vi "Teleop.vi"(10 "Match Info":T2={"Autonomous Elapsed Seconds"=0.0, "TeleOp Elapsed Seconds"=0.0, "Disabled Elapsed Seconds"=0.0, "Visited Autonomous"=FALSE, "Visited TeleOp"=FALSE, "Visited Disabled"=FALSE, "Autonomous Settings"={"Autonomous Style"=enum."Independent", "VI Refnum"=refnum}}, 11 "Call Context":T3) -> ()   [LabVIEW 2016]
doc: "This VI is called for each TeleOp packet received from the DS where the robot is not disabled. It is often used to read from the joysticks and update I/O or to update setpoints for timed control loops. It should complete and return within 20 milliseconds or it may miss DS packets."
uses:
  <vilib>/Rock Robotics/WPI/DriverStation/WPI_DriverStationDerivedRobotMode.ctl
  <vilib>/Rock Robotics/WPI/DriverStation/WPI_DriverStationMatch Info.ctl
  Robot Global Data.vi
  <vilib>/Rock Robotics/WPI/Utilities/WPI_GetSetVariantRefNum.vi
  <vilib>/Rock Robotics/WPI/Solenoid/Deprecated/WPI_SolenoidSetBool.vi
  <vilib>/Rock Robotics/Network Tables/NT Write Number.vi
  <vilib>/Rock Robotics/Network Tables/NT Write Boolean.vi
  <vilib>/addons/control/pid/pid.llb/PID (DBL).vi
  navX Library v2/navX Library v2.lvlib
  <vilib>/addons/control/pid/NI_PID_pid.lvlib
panel:
  in  "MOE":dbl=25.0 format="%#_13g"
  in  "Center":dbl=180.0 format="%#_13g"
  out "out left":dbl
  out "out right":dbl
  in  "Pid Factor":dbl=8400.0
  in  "Mode":bool=TRUE
  in  "output range":cluster{"output high":dbl, "output low":dbl}={"output high"=1.0, "output low"=-1.0} {"output low" format="%.2f"; "output high" format="%.2f"}
  in  "PID gains":T1={"proportional gain (Kc)"=0.00021, "integral time (Ti, min)"=15.0, "derivative time (Td, min)"=0.0} {"derivative time (Td, min)" format="%.6f"; "integral time (Ti, min)" format="%.6f"; "proportional gain (Kc)" format="%.6f"}
  out "Left":dbl(graph)
  out "Right":dbl(graph)
  out "Encoder Right":dbl(graph)
  out "Encoder Left":dbl(graph)
  in  "Speed":dbl=0.45 format="%#_13g"
  out "Out Left":dbl(graph)
  out "Out Right":dbl(graph)
  out "Shooter":cluster{"Sensor Velocity":dbl, dbl, dbl}(graph)
  in  "ShooterRPM":dbl
  in  "P":dbl=0.5 format="%#_13g"
  in  "I":dbl format="%#_13g"
  in  "D":dbl format="%#_13g"
  in  "F":dbl=0.005212 format="%#_13g"
  in  "I Zone":dbl format="%#_13g"
  in  "Ramp Rate":dbl format="%#_13g"
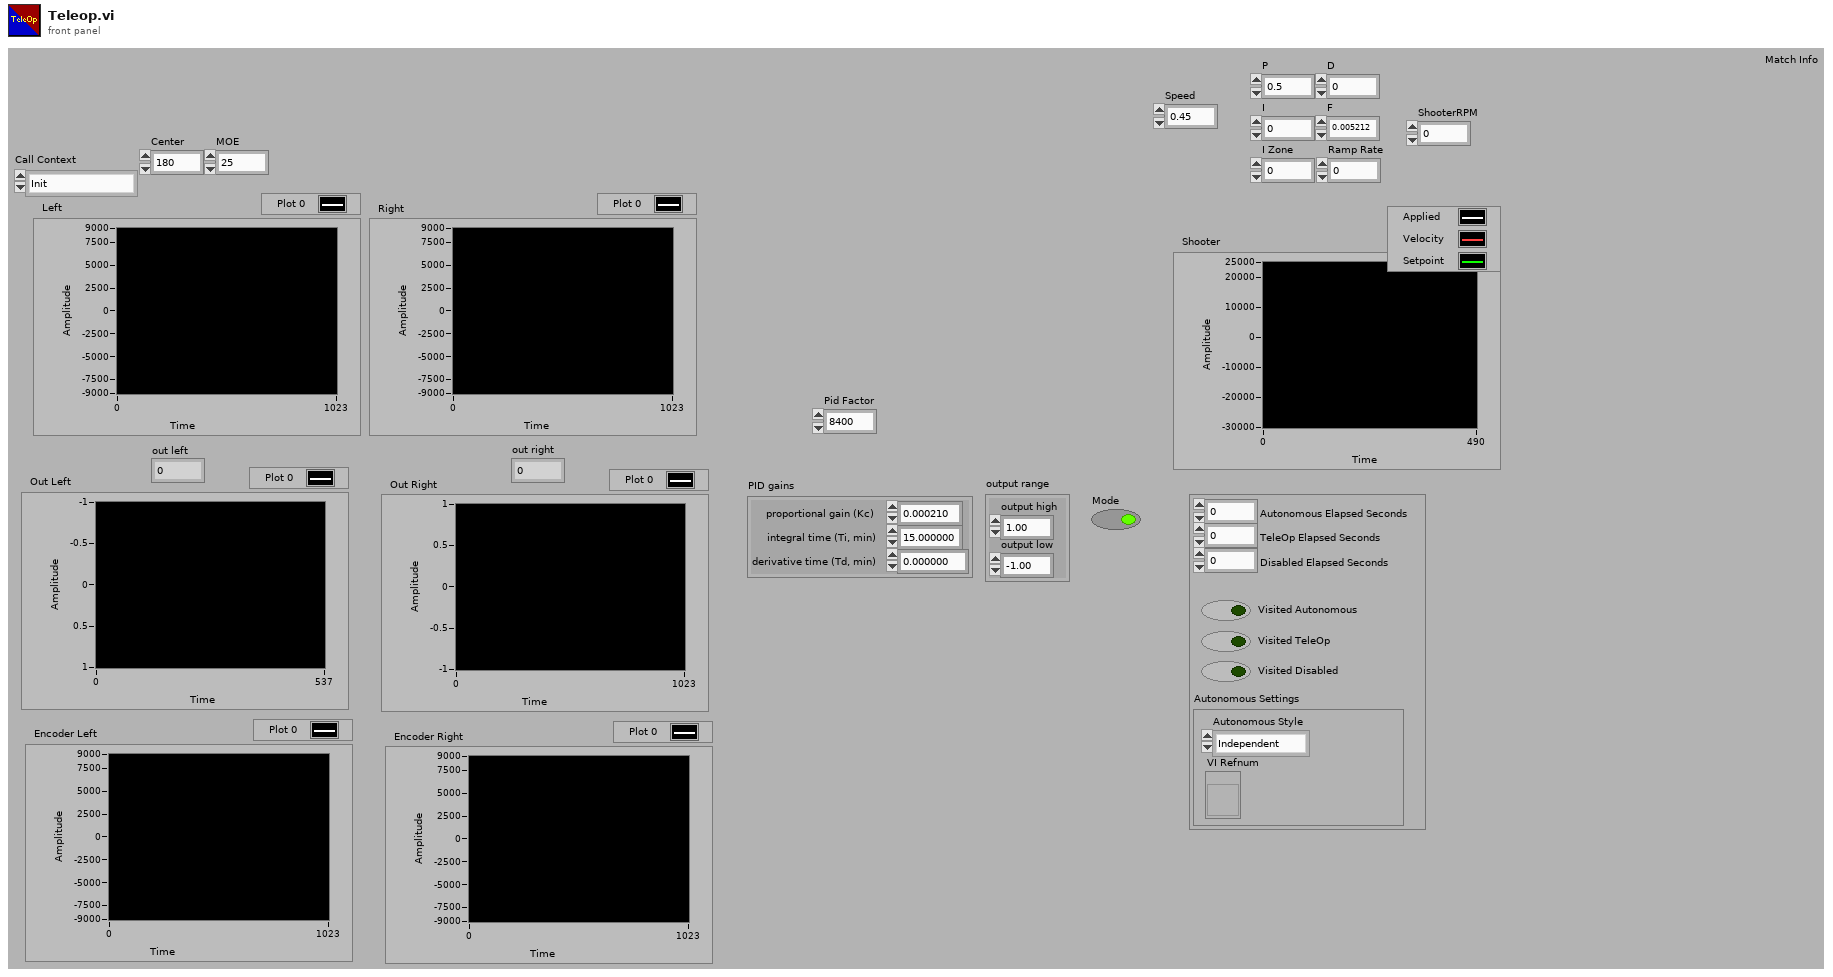
[diagram p1: front panel]
types:
  T1 = cluster{"proportional gain (Kc)":dbl, "integral time (Ti, min)":dbl, "derivative time (Td, min)":dbl}
  T2 = typedef "WPI_DriverStationMatch Info.ctl" = cluster{"Autonomous Elapsed Seconds":dbl, "TeleOp Elapsed Seconds":dbl, "Disabled Elapsed Seconds":dbl, "Visited Autonomous":bool, "Visited TeleOp":bool, "Visited Disabled":bool, "Autonomous Settings":cluster{"Autonomous Style":enum16{"Iterative", "Independent"}, "VI Refnum":refnum<vi>}}
  T3 = typedef "WPI_DriverStationDerivedRobotMode.ctl" = enum16{"Init", "Execute", "Stop"}
  T4 = typedef "WPI_SolenoidDevRef.ctl" = cluster{"DevStatus":errorcluster, "Pneumatics Control Module":u8, "Forward Solenoid Channel":T5, "Reverse Solenoid Channel":T5}
  T5 = typedef "WPI_SolenoidChannel.ctl" = enum8{"Solenoid 0", "Solenoid 1", "Solenoid 2", "Solenoid 3", "Solenoid 4", "Solenoid 5", "Solenoid 6", "Solenoid 7", "Invalid"}
  T6 = typedef "WPI_JoystickDevRef.ctl" = cluster{"Device":T7}
  T7 = typedef "WPI_JoystickDeviceEnum.ctl" = enum16{"USB 0", "USB 1", "USB 2", "USB 3", "USB 4", "USB 5"}
  T8 = cluster{"Buttons[0]":bool, "Buttons[1]":bool, "Buttons[2]":bool, "Buttons[3]":bool, "Buttons[4]":bool, "Buttons[5]":bool, "Buttons[6]":bool, "Buttons[7]":bool, "Buttons[8]":bool}
  T9 = cluster{"Axes[0]":dbl, "Axes[1]":dbl, "Axes[2]":dbl, "Axes[3]":dbl, "Axes[4]":dbl, "Axes[5]":dbl, "Axes[6]":dbl, "Axes[7]":dbl, "Axes[8]":dbl}
  T10 = typedef "navX Library v2.lvlib/Z900_navX_DeviceTypeDef.ctl" = cluster{"Interface":cluster{"Protocol":T11, "Update Rate (4Hz-100Hz)":u8, "navX Open TypeDef":variant}, "Notify Packet":refnum<notifier>, "Loop VI Refnum":refnum<vi>, "Ready to Close Occurrence Refnum":refnum<k4>}
  T11 = typedef "navX Library v2.lvlib/Z900_navX_ProtocolTypeDef.ctl" = enum16{"SERIAL", "I2C", "SPI"}
  T12 = cluster{"Velocity X":dbl, "Velocity Y":dbl, "Velocity Z":dbl, "Displacement X":dbl, "Displacement Y":dbl, "Displacement Z":dbl}
  T13 = cluster{"LinearAcceleration X":dbl, "LinearAcceleration Y":dbl, "LinearAcceleration Z":dbl}
  T14 = cluster{"Yaw":dbl, "Roll":dbl, "Pitch":dbl, "Heading":dbl, "Fused Heading":dbl}
  T15 = typedef "WPI_MotorControlDeviceRef.ctl" = cluster{"DeviceStatus":errorcluster, "Type":T16, "PWM":cluster{"PWM Channel":T17, "DeadBand":T18}, "CAN":cluster{"Device Number":u8, "SetOutput VI Ref":variant, "GetOutput VI Ref":variant, "Enable VI Ref":variant, "Disable VI Ref":variant, "Data":variant}, "Invert":bool}
  T16 = typedef "WPI_MotorControlType.ctl" = enum16{"PWM", "CAN"}
  T17 = typedef "FPGA_DIOPWMChannel.ctl" = enum8{"PWM 0", "PWM 1", "PWM 2", "PWM 3", "PWM 4", "PWM 5", "PWM 6", "PWM 7", "PWM 8", "PWM 9", "PWM MXP 0", "PWM MXP 1", "PWM MXP 2", "PWM MXP 3", "PWM MXP 4", "PWM MXP 5", "PWM MXP 6", "PWM MXP 7", "PWM MXP 8", "PWM MXP 9", "Invalid"}
  T18 = typedef "WPI_PWMDeadband.ctl" = cluster{"Name":string, "maxPositivePwm":i32, "minPositivePwm":i32, "centerPwm":i32, "maxNegativePwm":i32, "minNegativePwm":i32, "angularRange":u16}
  T19 = typedef "WPI_CANTalonSRX_GlobalStatus.ctl" = cluster{"Applied Throttle":dbl, "Module Enabled":bool, "CAN Error":errorcluster, "Closed Loop Error":dbl, "Forward Limit Switch Closed":bool, "Reverse Limit Switch Closed":bool, "Sensor Position":dbl, "Sensor Velocity":dbl, "Current":dbl, "Sticky Fault - Over Temp":bool, "Sticky Fault - Under Voltage":bool, "Sticky Fault - Forward Limit":bool, "Sticky Fault - Reverse Limit":bool, "Sticky Fault - Forward Soft Limit":bool, "Sticky Fault - Reverse Soft Limit":bool, "Brake is Enabled":bool, "Encoder Position":dbl, "Encoder Velocity":dbl, "Encoder Index Count":dbl, "Encoder A Pin State":bool, "Encoder B Pin State":bool, "Encoder Index Pin State":bool, "Analog In":dbl, "Analog In Velocity":dbl, "Temperature (C)":dbl, "Battery Voltage":dbl, "Control 5 Is Supported":bool, "Current Profile Slot Select":dbl, "Pos Div 8":bool, "Vel Div 4":bool, "Pulse Width Position":i32, "Pulse Width Velocity":i32, "Pulse Width Rise To Rise (us)":i32, "Pulse Width Rise To Fall (us)":i32, "Mot Prof Active Is Under Run":bool, "Mot Prof Active Has Under Run":bool, "Mot Prof Active Is Last":bool, "Mot Prof Active Velocity Only":bool, "Mot Prof Active Is Valid":bool, "Mot Prof Buffer Is Full":bool, "Mot Prof Active Profile Slot Select":i32, "Mot Prof NextID":i32, "Mot Prof Count":i32, "Mot Prof Active Velocity":dbl, "Mot Prof Active Position":dbl, "Mot Prof Output Enable":i32}
  T20 = cluster{dbl, "Sensor Velocity":dbl, "ShooterRPM":dbl}
  T21 = typedef "WPI_EncoderDevRef.ctl" = cluster{"DevStatus":errorcluster, "EncoderIndex":T22, "CounterIndex":T23, "DistancePerCount":dbl, "Decoding Type":T24}
  T22 = typedef "FPGA_EncoderIdx.ctl" = enum8{"Enc 0", "Enc 1", "Enc 2", "Enc 3", "Enc 4", "Enc 5", "Enc 6", "Enc 7", "Invalid"}
  T23 = typedef "FPGA_CounterCtrSystemIndex.ctl" = enum8{"Ctr 0", "Ctr 1", "Ctr 2", "Ctr 3", "Ctr 4", "Ctr 5", "Ctr 6", "Ctr 7", "Invalid"}
  T24 = typedef "WPI_EncoderType.ctl" = enum16{"1x", "2x", "4x"}
  T25 = typedef "WPI_RobotDriveDevRef.ctl" = cluster{"DevStatus":errorcluster, "Motors[]":T15[], "Square Inputs":bool, "Max Output":dbl}
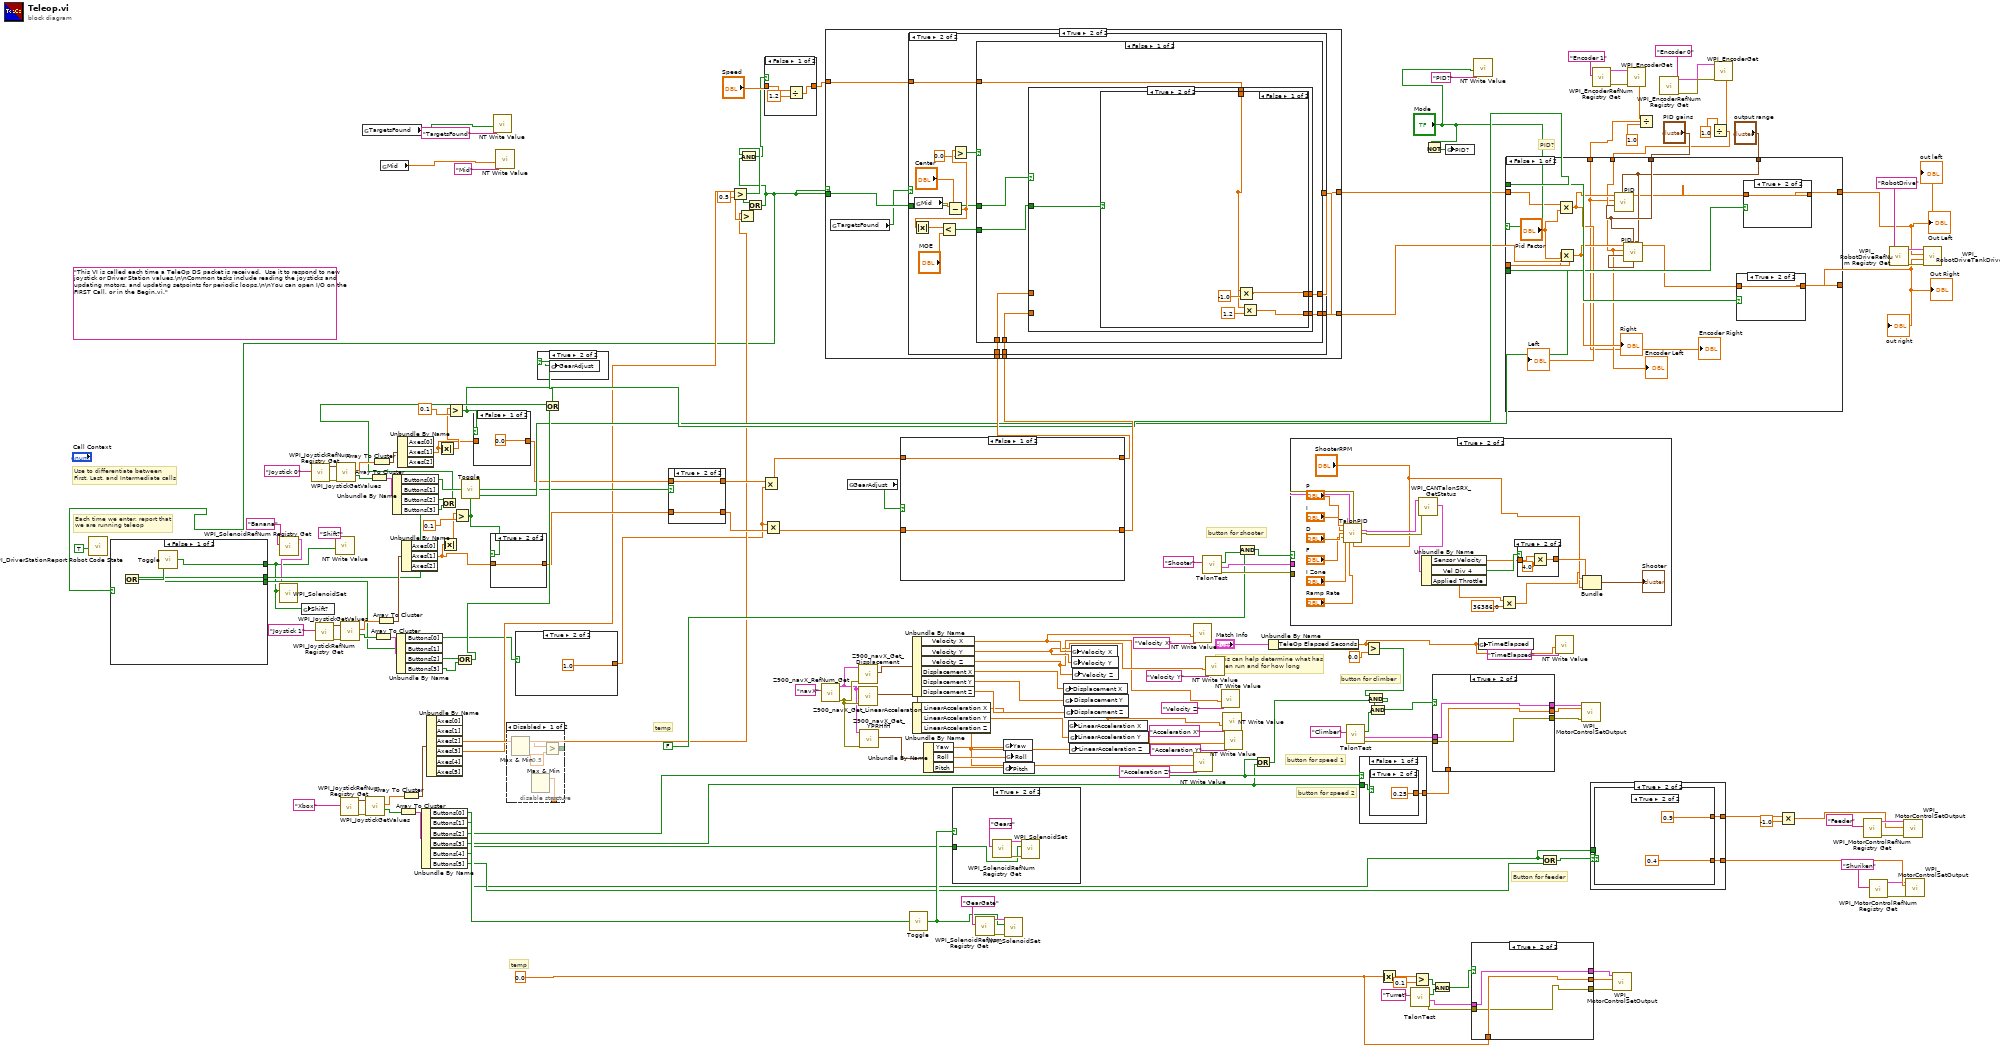
[diagram p0: block diagram]
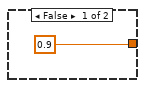
[diagram p2: hidden frame]
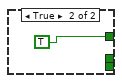
[diagram p3: hidden frame]
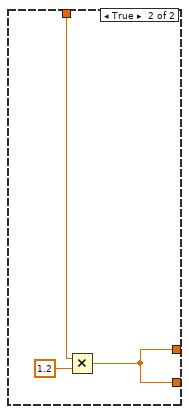
[diagram p8: hidden frame]
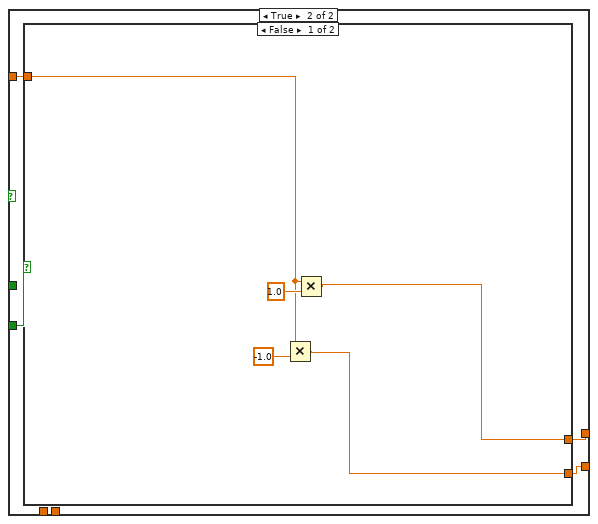
[diagram p9: hidden frame]
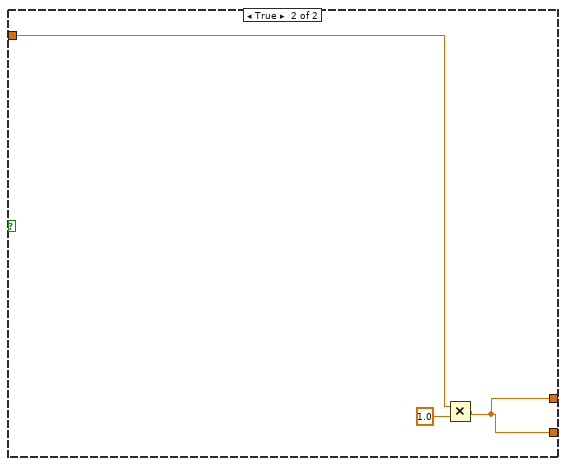
[diagram p10: hidden frame]
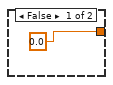
[diagram p11: hidden frame]
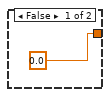
[diagram p12: hidden frame]
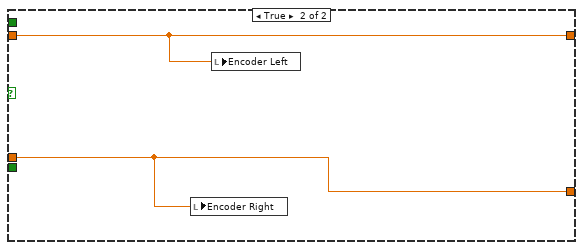
[diagram p13: hidden frame]
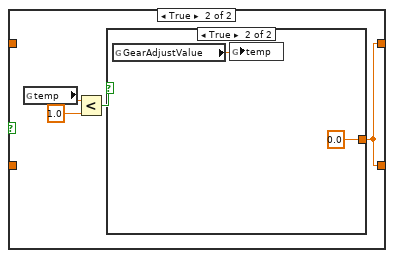
[diagram p16: hidden frame]
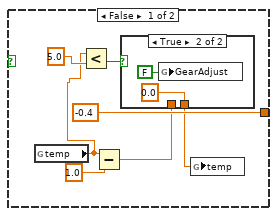
[diagram p17: hidden frame]
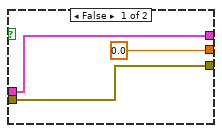
[diagram p19: hidden frame]
diagram:
  w38 = 0.5 ("y")
  w78 = 0.0
  (unwired) "This VI is called each time a TeleOp DS packet is received.  Use it to respond to new joystick or Driver Station values.\n\nCommon tasks include reading the joysticks and updating motors, and updating setpoints for periodic loops.\n\nYou can open I/O on the FIRST Call, or in the Begin.vi."
  # "PID?"
  # "temp"
  # "temp"
  # "Button for feeder"
  # "button for speed 2"
  # "button for speed 1"
  # "button for climber"
  # "button for shooter"
  # "Each time we enter, report that\nwe are running teleop"
  # "Use to differentiate between\nFirst, Last, and Intermediate calls"
  # "This can help determine what has\nbeen run and for how long"
  n1 = call <vilib>:"WPI_DriverStationReport Robot Code State.vi"("TeleOp"=TRUE ("Autonomous")) -> ()  [unwired: 10 in, 1 out]
  n2 = call <vilib>:"WPI_SolenoidRefNum Registry Get.vi"("refnum name"="Banana") -> ("SolenoidDevRef"=w8:T4)  [unwired: 9 in, 1 out]
  n3 = call <vilib>:"WPI_JoystickRefNum Registry Get.vi"("refnum name"="Joystick 0") -> ("error out"=w171:errorcluster, "JoystickDevRef"=w170:T6)  [unwired: 9 in]
  n4 = call <vilib>:"WPI_JoystickRefNum Registry Get.vi"("refnum name"="Joystick 1") -> ("error out"=w163:errorcluster, "JoystickDevRef"=w162:T6)  [unwired: 9 in]
  n5 = call <vilib>:"WPI_JoystickGetValues.vi"("error in (no error)"=w171, "JoystickDevRef"=w170) -> ("Buttons"=w167:bool[], "Axes"=w168:dbl[])  [unwired: 5 in, 3 out]
  n6 = call <vilib>:"WPI_JoystickRefNum Registry Get.vi"("refnum name"="Xbox") -> ("error out"=w125:errorcluster, "JoystickDevRef"=w124:T6)  [unwired: 9 in]
  n7 = call <vilib>:"WPI_JoystickGetValues.vi"("error in (no error)"=w163, "JoystickDevRef"=w162) -> ("Buttons"=w159:bool[], "Axes"=w160:dbl[])  [unwired: 5 in, 3 out]
  n8 = global read "Robot Global Data.vi" "TargetsFound"() -> (w12:bool)
  n9 = call <vilib>:"WPI_JoystickGetValues.vi"("error in (no error)"=w125, "JoystickDevRef"=w124) -> ("Buttons"=w121:bool[], "Axes"=w122:dbl[])  [unwired: 5 in, 3 out]
  n10 = Array To Cluster(array=w167) -> (cluster=w165:T8)
  n11 = Array To Cluster(array=w168) -> (cluster=w166:T9)
  n12 = Array To Cluster(array=w159) -> (cluster=w157:T8)
  n13 = Array To Cluster(array=w160) -> (cluster=w158:T9)
  n14 = global read "Robot Global Data.vi" "Mid"() -> (w10:dbl)
  n15 = Unbundle By Name(w165) -> ("Buttons[0]"=w151:bool, "Buttons[1]"=w41:bool, "Buttons[2]"=w84:bool, "Buttons[3]"=w83:bool)
  n16 = Unbundle By Name(w157) -> ("Buttons[0]"=w4:bool, "Buttons[1]"=w42:bool, "Buttons[2]"=w86:bool, "Buttons[3]"=w85:bool)
  n17 = Unbundle By Name(w166) -> ("Axes[1]"=w152:dbl)  [unwired: 2 out]
  n18 = Array To Cluster(array=w121) -> (cluster=w119:T8)
  n19 = Unbundle By Name(w158) -> ("Axes[1]"=w154:dbl)  [unwired: 2 out]
  n20 = Array To Cluster(array=w122) -> (cluster=w120:T9)
  n21 = Unbundle By Name(w119) -> ("Buttons[0]"=w118:bool, "Buttons[1]"=w117:bool, "Buttons[2]"=w116:bool, "Buttons[3]"=w115:bool, "Buttons[4]"=w112:bool, "Buttons[5]"=w113:bool)
  n22 = Unbundle By Name(w120) -> ("Axes[2]"=w32:dbl, "Axes[3]"=w31:dbl)  [unwired: 4 out]
  n23 = Absolute Value(x=w152) -> (abs(x)=w153:dbl)
  n24 = Or(x=w84, y=w83) -> (x .or. y?=w82:bool)
  n25 = Absolute Value(x=w154) -> (abs(x)=w155:dbl)
  n26 = Greater?(x=w153, y=0.1 ("x")) -> (0:w68:bool)
  n27 = Greater?(x=w155, y=0.1 ("x")) -> (0:w67:bool)
  n28 = Or(x=w86, y=w85) -> (x .or. y?=w81:bool)
  n29 = call "Toggle.vi"("Input"=w151) -> ("Output"=w62:bool)
  n30 = case shown="False" w68 {
    tunnel: w152 -> [_ w174]
    tunnel: [0.0 w174] -> w65
    frame False {
    }
    frame True {
    }
  }
  n31 = case shown="True" w67 {
    tunnel: w154 -> [_ w176]
    tunnel: [0.0 w176] -> w66
    frame False {
    }
    frame True {
    }
  }
  n32 = call-poly <vilib>:"NT Write Value.vi"("Boolean"=w12, "Name"="TargetsFound") -> ()  [unwired: 9 in, 1 out]
  n33 = call-poly <vilib>:"NT Write Value.vi"("Numeric"=w10, "Name"="Mid") -> ()  [unwired: 9 in, 1 out]
  n34 = disable-structure shown="Disabled" {
    disable-tunnel: [w178 _] -> _
    disable-tunnel: [w177 _] -> _
    frame Disabled {
      n35 = Max & Min() -> (max(x,y)=w180:dbl)  [unwired: 2 in, 1 out]
      n36 = Max & Min() -> (max(x,y)=w177:dbl)  [unwired: 2 in, 1 out]
      n37 = Greater?(x=w180, y=0.5) -> (0:w178:bool)
    }
    frame Enabled {
    }
  }
  n38 = case shown="True" w4 {
    tunnel: [0.9 1.0] -> w1
    frame False {
    }
    frame True {
    }
  }
  n39 = Or(x=w82, y=w81) -> (x .or. y?=w79:bool)
  n40 = case shown="True" w79 {
    selector: w79 -> [_ w183]
    frame False {
    }
    frame True {
      n41 = global write "Robot Global Data.vi" "GearAdjust"(w183) -> ()
    }
  }
  n42 = case shown="True" w62 {
    tunnel: w65 -> [w185 w190]
    tunnel: w66 -> [w184 w189]
    tunnel: [w188 w190] -> w64
    tunnel: [w187 w189] -> w63
    frame False {
      w186 = -1.0
      n43 = Multiply(x=w186, y=w185) -> (x*y=w187:dbl)
      n44 = Multiply(x=w184, y=w186) -> (x*y=w188:dbl)
    }
    frame True {
    }
  }
  n45 = Greater?(x=w31, y=w38) -> (0:w36:bool)
  n46 = Greater?(x=w32, y=w38) -> (0:w37:bool)
  n47 = Or(x=w36, y=w37) -> (x .or. y?=w7:bool)
  n48 = case shown="False" w7 {
    tunnel: w42 -> [w193 _]
    tunnel: w41 -> [w192 _]
    tunnel: [w191 TRUE] -> w5
    frame False {
      n49 = Or(x=w192, y=w193) -> (x .or. y?=w194:bool)
      n50 = call "Toggle.vi"("Input"=w194) -> ("Output"=w191:bool)
    }
    frame True {
    }
  }
  n51 = call-poly <vilib>:"WPI_SolenoidSet.vi"("Value"=w5, "SolenoidDevRef"=w8) -> ()  [unwired: 8 in, 2 out]
  n52 = global write "Robot Global Data.vi" "Shift?"(w5) -> ()
  n53 = call-poly <vilib>:"NT Write Value.vi"("Boolean"=w5, "Name"="Shift?") -> ()  [unwired: 9 in, 1 out]
  n54 = And(x=w36, y=w7) -> (x .and. y?=w33:bool)
  n55 = Multiply(x=w64, y=w1) -> (x*y=w3:dbl)
  n56 = case shown="False" w33 {
    tunnel: [w198 w199] -> w34
    tunnel: "Speed" -> [w197 w199]
    frame False {
      n57 = Divide(x=w197, y=1.2) -> (x/y=w198:dbl)
    }
    frame True {
    }
  }
  n58 = Multiply(x=w1, y=w63) -> (x*y=w2:dbl)
  n59 = call "Z900_navX_RefNum_Get.vi"("refnum name"="navX") -> ("error out"=w149:errorcluster, "navX Device"=w148:T10)  [unwired: 9 in]
  n60 = global read "Robot Global Data.vi" "GearAdjust"() -> (w80:bool)
  n61 = call "Z900_navX_Get_Displacement.vi"("error in (no error)"=w149, "navX Device"=w148) -> ("Displacement"=w145:T12)  [unwired: 6 in, 3 out]
  n62 = call "Z900_navX_Get_LinearAcceleration.vi"("error in (no error)"=w149, "navX Device"=w148) -> ("Linear Acceleration"=w146:T13)  [unwired: 6 in, 3 out]
  n63 = call "Z900_navX_Get_YPRHfH.vi"("error in (no error)"=w149, "navX Device"=w148) -> ("YRPHfH"=w147:T14)  [unwired: 6 in, 3 out]
  n64 = case shown="False" w80 {
    tunnel: w3 -> [w201 _]
    tunnel: w2 -> [w200 _]
    tunnel: [w201 w202] -> w73
    tunnel: [w200 w202] -> w72
    frame False {
    }
    frame True {
      n65 = global read "Robot Global Data.vi" "temp"() -> (w205:dbl)
      n66 = Less?(x=w205, y=1.0) -> (x < y?=w203:bool)
      n67 = case shown="True" w203 {
        tunnel: [-0.4 0.0] -> w202
        frame False {
          n68 = global read "Robot Global Data.vi" "temp"() -> (w208:dbl)
          n69 = Less?(x=w208, y=5.0 ("x")) -> (x < y?=w209:bool)
          n70 = Subtract(x=w208, y=1.0) -> (x-y=w206:dbl)
          n71 = case shown="True" w209 {
            tunnel: [w213 0.0] -> w207
            tunnel: w206 -> [w213 _]
            frame False {
            }
            frame True {
              n72 = global write "Robot Global Data.vi" "GearAdjust"(FALSE) -> ()
            }
          }
          n73 = global write "Robot Global Data.vi" "temp"(w207) -> ()
        }
        frame True {
          n74 = global read "Robot Global Data.vi" "GearAdjustValue"() -> (w217:dbl)
          n75 = global write "Robot Global Data.vi" "temp"(w217) -> ()
        }
      }
    }
  }
  n76 = case shown="True" w7 {
    tunnel: w73 -> [w219 w226]
    tunnel: w72 -> [w218 w225]
    tunnel: w7 -> [_ w224]
    tunnel: [w219 w220] -> w39
    tunnel: [w218 w221] -> w40
    tunnel: w34 -> [_ w222]
    frame False {
    }
    frame True {
      n77 = global read "Robot Global Data.vi" "TargetsFound"() -> (w223:bool)
      n78 = case shown="True" w223 {
        tunnel: w226 -> [w227 w237]
        tunnel: w225 -> [w228 w236]
        tunnel: [w227 w235] -> w220
        tunnel: [w228 w234] -> w221
        tunnel: w224 -> [_ w230]
        tunnel: w222 -> [_ w229]
        frame False {
        }
        frame True {
          n79 = global read "Robot Global Data.vi" "Mid"() -> (w242:dbl)
          n80 = Subtract(x=w242, y="Center") -> (x-y=w232:dbl)
          n81 = Absolute Value(x=w232) -> (abs(x)=w240:dbl)
          n82 = Less?(x=w240, y="MOE") -> (x < y?=w238:bool)
          n83 = Greater?(x=w232, y=0.0) -> (0:w233:bool)
          n84 = case shown="False" w233 {
            tunnel: w238 -> [w249 w267]
            tunnel: w237 -> [w248 _]
            tunnel: w236 -> [w247 _]
            tunnel: [w246 w265] -> w235
            tunnel: [w245 w266] -> w234
            tunnel: w230 -> [w244 _]
            tunnel: w229 -> [w243 w264]
            frame False {
              n85 = case shown="True" w244 {
                tunnel: w249 -> [_ w255]
                tunnel: w248 -> [w251 _]
                tunnel: w247 -> [w250 _]
                tunnel: [w251 w254] -> w245
                tunnel: [w250 w253] -> w246
                tunnel: w243 -> [_ w252]
                frame False {
                }
                frame True {
                  n86 = case shown="False" w255 {
                    tunnel: [w260 w263] -> w254
                    tunnel: [w258 w263] -> w253
                    tunnel: w252 -> [w256 w261]
                    frame False {
                      n87 = Multiply(x=w256, y=-1.0) -> (x*y=w260:dbl)
                      n88 = Multiply(x=w256, y=1.2) -> (x*y=w258:dbl)
                    }
                    frame True {
                      n89 = Multiply(x=w261, y=1.2) -> (x*y=w263:dbl)
                    }
                  }
                }
              }
            }
            frame True {
              n90 = case shown="False" w267 {
                tunnel: [w272 w275] -> w266
                tunnel: [w270 w275] -> w265
                tunnel: w264 -> [w268 w273]
                frame False {
                  n91 = Multiply(x=w268, y=-1.0) -> (x*y=w270:dbl)
                  n92 = Multiply(x=w268, y=1.0) -> (x*y=w272:dbl)
                }
                frame True {
                  n93 = Multiply(x=w273, y=1.0) -> (x*y=w275:dbl)
                }
              }
            }
          }
        }
      }
    }
  }
  n94 = call "Toggle.vi"("Input"=w118) -> ("Output"=w126:bool)
  n95 = Unbundle By Name(w145) -> ("Velocity X"=w19:dbl, "Velocity Y"=w18:dbl, "Velocity Z"=w17:dbl, "Displacement X"=w61:dbl, "Displacement Y"=w60:dbl, "Displacement Z"=w59:dbl)
  n96 = Unbundle By Name(w146) -> ("LinearAcceleration X"=w16:dbl, "LinearAcceleration Y"=w15:dbl, "LinearAcceleration Z"=w14:dbl)
  n97 = Unbundle By Name(w147) -> ("Yaw"=w58:dbl, "Roll"=w57:dbl, "Pitch"=w56:dbl)
  n98 = case shown="True" w126 {
    tunnel: w117 -> [_ w276]
    frame False {
    }
    frame True {
      n99 = call <vilib>:"WPI_SolenoidRefNum Registry Get.vi"("refnum name"="Gears") -> ("error out"=w279:errorcluster, "SolenoidDevRef"=w278:T4)  [unwired: 9 in]
      n100 = call-poly <vilib>:"WPI_SolenoidSet.vi"("error in (no error)"=w279, "Value"=w276, "SolenoidDevRef"=w278) -> ()  [unwired: 7 in, 2 out]
    }
  }
  n101 = call <vilib>:"WPI_SolenoidRefNum Registry Get.vi"("refnum name"="GearGate") -> ("error out"=w129:errorcluster, "SolenoidDevRef"=w128:T4)  [unwired: 9 in]
  n102 = global write "Robot Global Data.vi" "Pitch"(w56) -> ()
  n103 = global write "Robot Global Data.vi" "Yaw"(w58) -> ()
  n104 = call-poly <vilib>:"WPI_SolenoidSet.vi"("error in (no error)"=w129, "Value"=w126, "SolenoidDevRef"=w128) -> ()  [unwired: 7 in, 2 out]
  n105 = global write "Robot Global Data.vi" "Roll"(w57) -> ()
  n106 = global write "Robot Global Data.vi" "Displacement X"(w61) -> ()
  n107 = global write "Robot Global Data.vi" "Displacement Y"(w60) -> ()
  n108 = global write "Robot Global Data.vi" "Displacement Z"(w59) -> ()
  n109 = global write "Robot Global Data.vi" "LinearAcceleration X"(w16) -> ()
  n110 = global write "Robot Global Data.vi" "LinearAcceleration Y"(w15) -> ()
  n111 = global write "Robot Global Data.vi" "LinearAcceleration Z"(w14) -> ()
  n112 = global write "Robot Global Data.vi" "Velocity X"(w19) -> ()
  n113 = global write "Robot Global Data.vi" "Velocity Y"(w18) -> ()
  n114 = global write "Robot Global Data.vi" "Velocity Z"(w17) -> ()
  n115 = call-poly <vilib>:"NT Write Value.vi"("Numeric"=w19, "Name"="Velocity X") -> ()  [unwired: 9 in, 1 out]
  n116 = call-poly <vilib>:"NT Write Value.vi"("Numeric"=w14, "Name"="Acceleration Z") -> ()  [unwired: 9 in, 1 out]
  n117 = call "TalonTest.vi"("Name"="Shooter") -> ("Output"=w139:bool, "Ref"=w143:T15, "error out"=w142:errorcluster)  [unwired: 7 in]
  n118 = call-poly <vilib>:"NT Write Value.vi"("Numeric"=w18, "Name"="Velocity Y") -> ()  [unwired: 9 in, 1 out]
  n119 = call-poly <vilib>:"NT Write Value.vi"("Numeric"=w17, "Name"="Velocity Z") -> ()  [unwired: 9 in, 1 out]
  n120 = call-poly <vilib>:"NT Write Value.vi"("Numeric"=w16, "Name"="Acceleration X") -> ()  [unwired: 9 in, 1 out]
  n121 = call-poly <vilib>:"NT Write Value.vi"("Numeric"=w15, "Name"="Acceleration Y") -> ()  [unwired: 9 in, 1 out]
  n122 = And(x=FALSE, y=w139) -> (x .and. y?=w140:bool)
  n123 = Or(x=w116, y=w115) -> (x .or. y?=w114:bool)
  n124 = Unbundle By Name("Match Info") -> ("TeleOp Elapsed Seconds"=w29:dbl)
  n125 = case shown="True" w140 {
    tunnel: w143 -> [_ w284]
    tunnel: w142 -> [_ w280]
    frame False {
    }
    frame True {
      n126 = call "TalonPID.vi"("P"="P", "Ref In"=w284, "Error in"=w280, "I"="I", "D"="D", "F"="F", "I Zone"="I Zone", "Ramp Rate"="Ramp Rate", "Output"="ShooterRPM") -> ("Ref Out"=w283:T15, "error out"=w282:errorcluster)  [unwired: 5 in]
      n127 = call <vilib>:"WPI_CANTalonSRX_GetStatus.vi"("error in (no error)"=w282, "CAN Talon SRX Ref"=w283) -> ("Talon SRX Status"=w298:T19)  [unwired: 7 in, 2 out]
      n128 = Unbundle By Name(w298) -> ("Sensor Velocity"=w296:dbl, "Vel Div 4"=w297:bool, "Applied Throttle"=w293:dbl)
      n129 = Multiply(x=w293, y=36386.0) -> (x*y=w292:dbl)
      n130 = case shown="True" w297 {
        tunnel: w296 -> [w299 w301]
        tunnel: [w299 w302] -> w291
        frame False {
        }
        frame True {
          n131 = Multiply(x=w301, y=4.0) -> (x*y=w302:dbl)
        }
      }
      n132 = Bundle(w292, "Sensor Velocity"=w291, "ShooterRPM"="ShooterRPM") -> (→"Shooter":T20)  [unwired: 1 in]
    }
  }
  n133 = call "TalonTest.vi"("Name"="Climber") -> ("Output"=w137:bool, "Ref"=w132:T15, "error out"=w131:errorcluster)  [unwired: 7 in]
  n134 = case shown="False" w116 {
    tunnel: [w304 w308] -> w130
    tunnel: w115 -> [w303 w307]
    frame False {
      n135 = case shown="True" w303 {
        tunnel: [0.0 0.25] -> w304
        frame False {
        }
        frame True {
        }
      }
    }
    frame True {
      n136 = case shown="True" w307 {
        tunnel: [0.75 1.0] -> w308
        frame False {
        }
        frame True {
        }
      }
    }
  }
  n137 = Greater?(x=w29, y=0.0) -> (0:w134:bool)
  n138 = And(x=w134, y=w114) -> (x .and. y?=w138:bool)
  n139 = And(x=w138, y=w137) -> (x .and. y?=w133:bool)
  n140 = Absolute Value(x=w78) -> (abs(x)=w105:dbl)
  n141 = call "TalonTest.vi"("Name"="Turret") -> ("Output"=w109:bool, "Ref"=w107:T15, "error out"=w106:errorcluster)  [unwired: 7 in]
  n142 = Greater?(x=w105, y=0.1) -> (0:w103:bool)
  n143 = Not(x="Mode") -> (.not. x?=w30:bool)
  n144 = case shown="True" w133 {
    tunnel: w132 -> [w312 w316]
    tunnel: w131 -> [w311 w314]
    tunnel: w130 -> [_ w315]
    tunnel: [w312 w316] -> w98
    tunnel: [0.0 w315] -> w99
    tunnel: [w311 w314] -> w97
    frame False {
    }
    frame True {
    }
  }
  n145 = And(x=w103, y=w109) -> (x .and. y?=w108:bool)
  n146 = global write "Robot Global Data.vi" "PID?"(w30) -> ()
  n147 = case shown="True" w108 {
    tunnel: w107 -> [w318 w322]
    tunnel: w106 -> [w317 w320]
    tunnel: w78 -> [_ w321]
    tunnel: [w318 w322] -> w102
    tunnel: [0.0 w321] -> w101
    tunnel: [w317 w320] -> w100
    frame False {
    }
    frame True {
    }
  }
  n148 = call-poly <vilib>:"NT Write Value.vi"("Boolean"="Mode", "Name"="PID?") -> ()  [unwired: 9 in, 1 out]
  n149 = global write "Robot Global Data.vi" "TimeElapsed"(w29) -> ()
  n150 = Or(x=w112, y=w113) -> (x .or. y?=w111:bool)
  n151 = call-poly <vilib>:"NT Write Value.vi"("Numeric"=w29, "Name"="TimeElapsed") -> ()  [unwired: 9 in, 1 out]
  n152 = call <vilib>:"WPI_MotorControlSetOutput.vi"("error in (no error)"=w97, "Output"=w99, "MotorControlDevRef"=w98) -> ()  [unwired: 6 in, 3 out]
  n153 = case shown="True" w111 {
    tunnel: w112 -> [_ w326]
    tunnel: [w323 w325] -> w89
    tunnel: [w323 w324] -> w96
    frame False {
      w323 = 0.0
    }
    frame True {
      n154 = case shown="True" w326 {
        tunnel: [-0.9 ("Output") 0.9 ("Output")] -> w325
        tunnel: [-0.4 ("Output") 0.4 ("Output")] -> w324
        frame False {
        }
        frame True {
        }
      }
    }
  }
  n155 = call <vilib>:"WPI_EncoderRefNum Registry Get.vi"("refnum name"="Encoder 1") -> ("error out"=w55:errorcluster, "EncoderDevRef"=w54:T21)  [unwired: 9 in]
  n156 = call <vilib>:"WPI_MotorControlSetOutput.vi"("error in (no error)"=w100, "Output"=w101, "MotorControlDevRef"=w102) -> ()  [unwired: 6 in, 3 out]
  n157 = call <vilib>:"WPI_EncoderGet.vi"("error in (no error)"=w55, "EncoderDevRef"=w54) -> ("Rate"=w45:dbl)  [unwired: 4 in, 5 out]
  n158 = Divide(x=w45, y=1.0) -> (x/y=w48:dbl)
  n159 = call <vilib>:"WPI_EncoderRefNum Registry Get.vi"("refnum name"="Encoder 0") -> ("error out"=w52:errorcluster, "EncoderDevRef"=w51:T21)  [unwired: 9 in]
  n160 = call <vilib>:"WPI_EncoderGet.vi"("error in (no error)"=w52, "EncoderDevRef"=w51) -> ("Rate"=w47:dbl)  [unwired: 4 in, 5 out]
  n161 = Divide(x=w47, y=1.0) -> (x/y=w49:dbl)
  n162 = case shown="False" "Mode" {
    tunnel: w39 -> [w336 w351]
    tunnel: w40 -> [w335 w350]
    tunnel: w48 -> [w331 _]
    tunnel: w49 -> [w332 _]
    tunnel: "PID gains" -> [w345 _]
    tunnel: "output range" -> [w344 _]
    tunnel: w68 -> [w341 _]
    tunnel: w67 -> [w340 _]
    tunnel: [w342 w350] -> w70
    tunnel: [w343 w351] -> w43
    frame False {
      n163 = Multiply(x=w336, y="Pid Factor") -> (x*y=w333:dbl)
      "Left" <- w333
      n164 = Multiply(x=w335, y="Pid Factor") -> (x*y=w334:dbl)
      "Right" <- w334
      n165 = call-poly <vilib>:"PID.vi"("output range"=w344, "PID gains"=w345, "process variable"=w331, "setpoint"=w333) -> ("output"=w339:dbl)  [unwired: 6 in, 1 out]
      n166 = call-poly <vilib>:"PID.vi"("output range"=w344, "PID gains"=w345, "process variable"=w332, "setpoint"=w334) -> ("output"=w338:dbl)  [unwired: 6 in, 1 out]
      n167 = case shown="True" w341 {
        tunnel: w338 -> [_ w347]
        tunnel: [0.0 w347] -> w342
        frame False {
        }
        frame True {
        }
      }
      n168 = case shown="True" w340 {
        tunnel: w339 -> [_ w349]
        tunnel: [0.0 w349] -> w343
        frame False {
        }
        frame True {
        }
      }
      "Encoder Right" <- w331
      "Encoder Left" <- w332
    }
    frame True {
      n169 = local write "Encoder Right"(w350) -> ()
      n170 = local write "Encoder Left"(w351) -> ()
    }
  }
  "Out Right" <- w70
  "Out Left" <- w43
  "out right" <- w70
  "out left" <- w43
  n171 = Multiply(x=w89, y=-1.0) -> (x*y=w87:dbl)
  n172 = call <vilib>:"WPI_MotorControlRefNum Registry Get.vi"("refnum name"="Feeder") -> ("error out"=w90:errorcluster, "MotorControlDevRef"=w91:T15)  [unwired: 9 in]
  n173 = call <vilib>:"WPI_MotorControlRefNum Registry Get.vi"("refnum name"="Shuriken") -> ("error out"=w92:errorcluster, "MotorControlDevRef"=w93:T15)  [unwired: 9 in]
  n174 = call <vilib>:"WPI_RobotDriveRefNum Registry Get.vi"("refnum name"="RobotDrive") -> ("error out"=w76:errorcluster, "RobotDriveDevRef"=w75:T25)  [unwired: 9 in]
  n175 = call <vilib>:"WPI_MotorControlSetOutput.vi"("error in (no error)"=w90, "Output"=w87, "MotorControlDevRef"=w91) -> ()  [unwired: 6 in, 3 out]
  n176 = call <vilib>:"WPI_MotorControlSetOutput.vi"("error in (no error)"=w92, "Output"=w96, "MotorControlDevRef"=w93) -> ()  [unwired: 6 in, 3 out]
  n177 = call <vilib>:"WPI_RobotDriveTankDrive.vi"("error in (no error)"=w76, "Right axis value"=w70, "Left axis value"=w43, "RobotDriveDevRef"=w75) -> ()  [unwired: 5 in, 3 out]
